vi "Set Voltage.vi"(0 "object in":refnum<class "PowerModuleInterface.lvclass">, 5 "voltage (V)":dbl, 11 "Error In":errorcluster) -> (4 "object out":refnum<class "PowerModuleInterface.lvclass">, 15 "Error Out":errorcluster)   [LabVIEW 2023, in "PowerModuleInterface.lvlib" / "PowerModuleInterface.lvclass"]
uses:
  PowerModuleInterface.lvclass
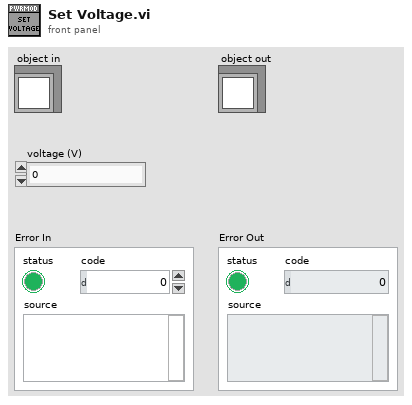
[diagram p1: front panel]
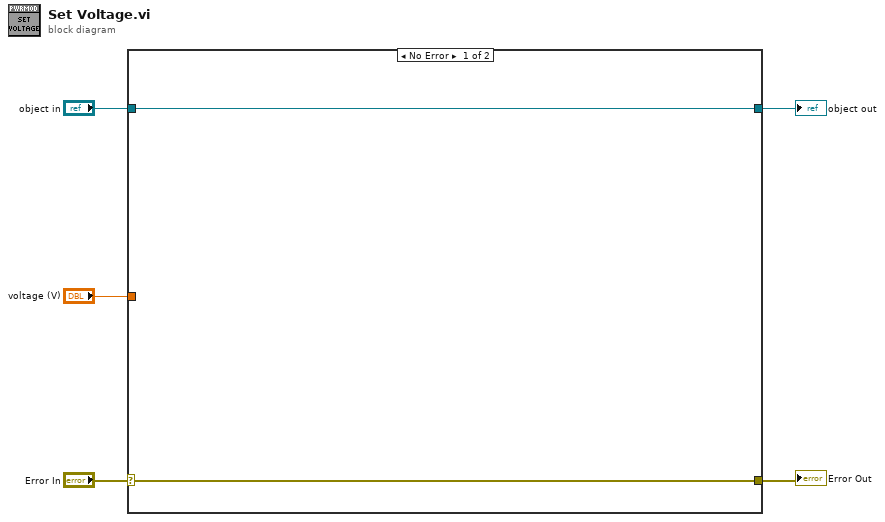
[diagram p0: block diagram]
diagram:
  n1 = case shown="No Error" "Error In" {
    selector: "Error In" -> [w7 w9]
    tunnel: [w7 w9] -> w4
    tunnel: [w6 w8] -> w2
    tunnel: "object in" -> [w6 w8]
    tunnel: "voltage (V)" -> [_ _]
    frame No Error {
    }
    frame Error {
    }
  }
  "Error Out" <- w4
  "object out" <- w2
